vi "Open Hardware.vi"(8 "error in (no error)":errorcluster, 11 "Instrument.FrameworkTemplate":refnum<class "Temperhum.PCSensor.lvclass">) -> (0 "error out":errorcluster, 3 "Instrument.FrameworkTemplate out":refnum<class "Temperhum.PCSensor.lvclass">)   [LabVIEW 2019, in "Temperhum.PCSensor.lvclass"]
uses:
  Temperhum.PCSensor.lvclass
  Temperhum.PCSensor.lvclass/Temperhum.PCSensor.ctl
  Instrument.Temperhum/Instrument.Temperhum.lvclass
  drivers/TEMPerHUM/RDingUSB.dll
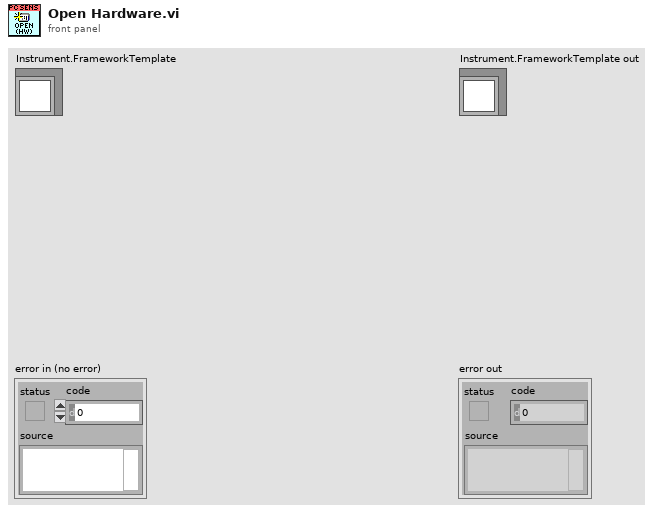
[diagram p1: front panel]
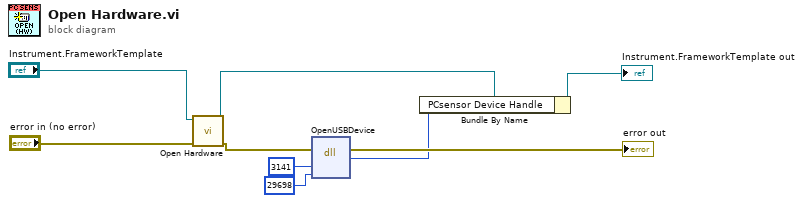
[diagram p0: block diagram]
diagram:
  n1 = call-parent "Open Hardware.vi"("error in (no error)"="error in (no error)", "Instrument.FrameworkTemplate"="Instrument.FrameworkTemplate") -> ("error out"=w3:errorcluster, "Instrument.FrameworkTemplate out"=w7:refnum<class "Temperhum.PCSensor.lvclass">)  [unwired: 8 in]
  n2 = dll-call lib="C:/Users/ansom/Documents/GitHub/Temperhum-Instrument/lvsrc/drivers/TEMPerHUM/RDingUSB.dll" fn="OpenUSBDevice"(error in=w3, "VID"=3141, "PID"=29698) -> (error out=→"error out":errorcluster, "return type"=w1:i64)  [unwired: 4 in, 1 out]
  n3 = Bundle By Name(cluster=w7, "PCsensor Device Handle"=w1) -> (→"Instrument.FrameworkTemplate out":refnum<class "Temperhum.PCSensor.lvclass">)
